vi "SinCos3.vi"() -> (8 "SinCos3":refnum<class "SinCos3.lvclass">)   [LabVIEW 2017, in "SinCos3.lvclass"]
uses:
  SinCos3.lvclass
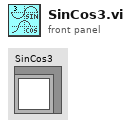
[diagram p1: front panel]
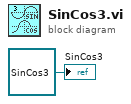
[diagram p0: block diagram]
diagram:
  "SinCos3" <- refnum<class "SinCos3.lvclass"> refnum ("SinCos3.lvclass")
